vi "Configure ADCW.vi"(0 "VISA resource name":refnum<visa-resource-name>, 1 "Test Voltage (V)":string, 2 "Ramp Time (s)":string, 3 "Dwell Time (s)":string, 4 "Min Leakag (A)":string, 5 "Max Leakage (A)":string, 6 "DUT Type I":string(combo)="Isolated DUT", 7 "error in (no error)":errorcluster, 8 "Test Mode":string(combo)="ACW", 9 "DUT Type II (DCW Only)":string(combo)="Resistive DUT", 11 "Command Terminator":bool=TRUE) -> (20 "VISA resource name out":refnum<visa-resource-name>, 21 "Command Output":string, 25 "Error Message":string, 26 "Error Code":i32, 27 "error out":errorcluster)   [LabVIEW 2010, in "VITREK V7X.lvlib"]
doc: "Configures the <b>ACW</b> or <b>DCW</b> input.\n\n<b>Note:</b> please refer to the instrument manual for the <b>ACW/DCW</b> input specification."
uses:
  VITREK V7X.lvlib
panel:
  # "Yes\n\nNo"
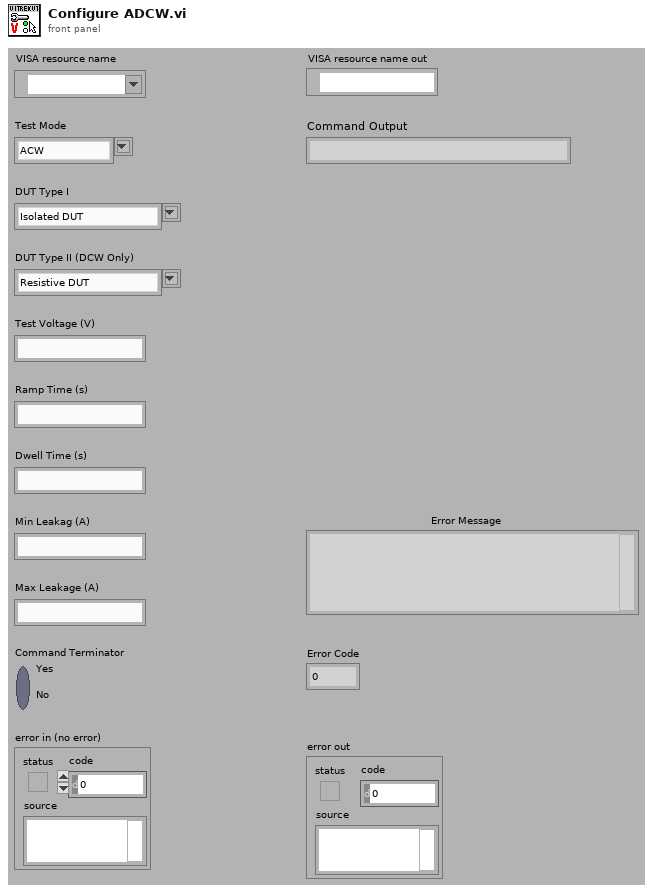
[diagram p1: front panel]
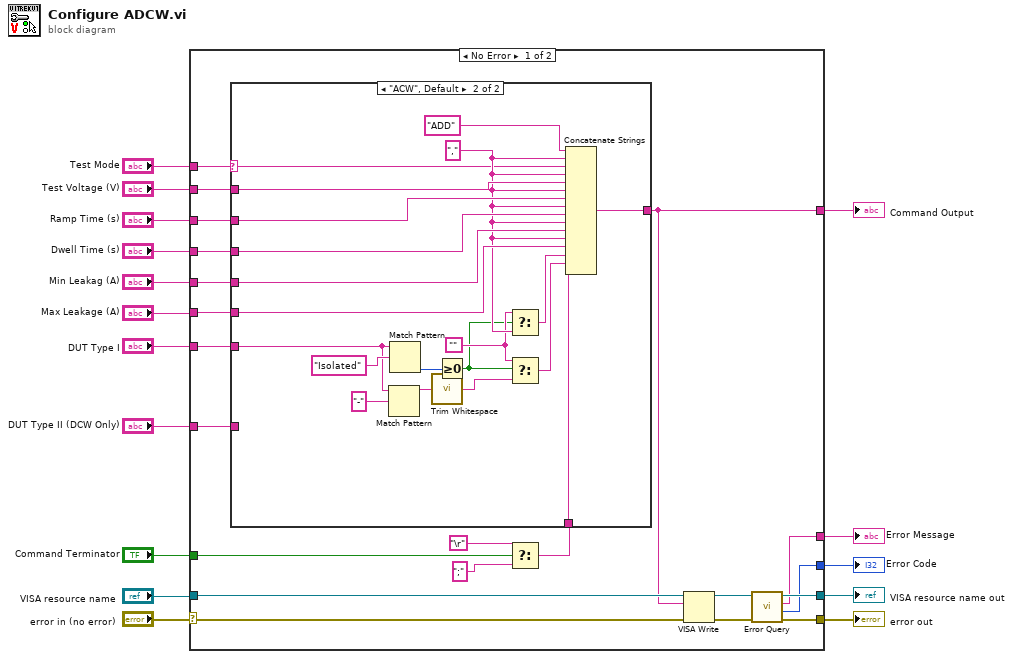
[diagram p0: block diagram]
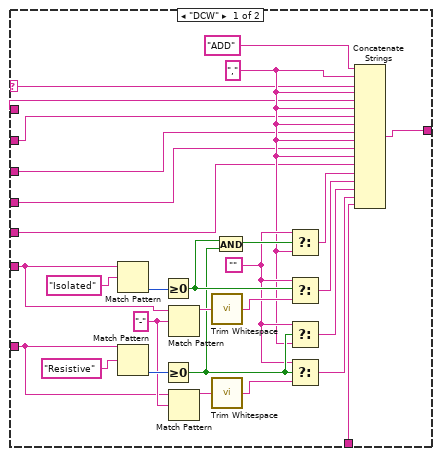
[diagram p2: hidden frame]
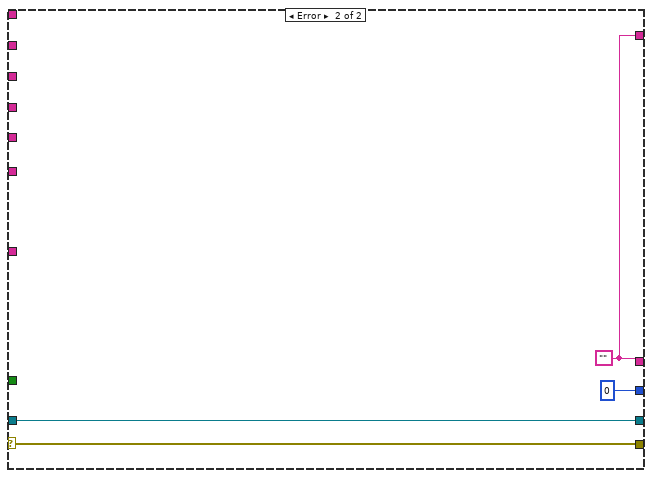
[diagram p3: hidden frame]
diagram:
  n1 = case shown="No Error" "error in (no error)" {
    selector: "error in (no error)" -> [w33 w89]
    tunnel: "VISA resource name" -> [w37 w90]
    tunnel: [w27 w87] -> w15
    tunnel: [w34 w90] -> w14
    tunnel: [w19 w89] -> w13
    tunnel: "Test Voltage (V)" -> [w32 _]
    tunnel: "Ramp Time (s)" -> [w31 _]
    tunnel: "Dwell Time (s)" -> [w30 _]
    tunnel: "Min Leakag (A)" -> [w29 _]
    tunnel: "Max Leakage (A)" -> [w28 _]
    tunnel: "Command Terminator" -> [w26 _]
    tunnel: "Test Mode" -> [w21 _]
    tunnel: "DUT Type I" -> [w22 _]
    tunnel: "DUT Type II (DCW Only)" -> [w20 _]
    tunnel: [w18 0 ("Error Code")] -> w2
    tunnel: [w17 w87] -> w1
    frame No Error {
      n2 = Select(t="\r", s=w26, f=";") -> (s? t:f=w23:string)
      n3 = case shown="\"ACW\", Default" w21 {
        selector: w21 -> [w47 w67]
        tunnel: w32 -> [w46 w86]
        tunnel: w31 -> [w45 w85]
        tunnel: w30 -> [w44 w84]
        tunnel: w29 -> [w43 w83]
        tunnel: w28 -> [w42 w82]
        tunnel: [w38 w80] -> w27
        tunnel: w23 -> [w39 w75]
        tunnel: w22 -> [w41 w70]
        tunnel: w20 -> [w40 _]
        frame "DCW" {
          w48 = "-"
          w51 = ""
          w50 = ","
          n4 = Match Pattern(string=w41, regular expression="Isolated") -> (offset past match=w62:i32)  [unwired: 1 in, 3 out]
          n5 = Match Pattern(string=w40, regular expression="Resistive") -> (offset past match=w58:i32)  [unwired: 1 in, 3 out]
          n6 = Greater Or Equal To 0?(x=w62) -> (x >= 0?=w55:bool)
          n7 = Greater Or Equal To 0?(x=w58) -> (x >= 0?=w52:bool)
          n8 = Match Pattern(string=w41, regular expression=w48) -> (before substring=w61:string)  [unwired: 1 in, 3 out]
          n9 = Match Pattern(string=w40, regular expression=w48) -> (before substring=w57:string)  [unwired: 1 in, 3 out]
          n10 = call <vilib>:"Trim Whitespace.vi"("string"=w61) -> ("trimmed string"=w60:string)  [unwired: 1 in]
          n11 = call <vilib>:"Trim Whitespace.vi"("string"=w57) -> ("trimmed string"=w56:string)  [unwired: 1 in]
          n12 = And(x=w55, y=w52) -> (x .and. y?=w54:bool)
          n13 = Select(t=w51, s=w54, f=w50) -> (s? t:f=w64:string)
          n14 = Select(t=w51, s=w55, f=w60) -> (s? t:f=w65:string)
          n15 = Select(t=w51, s=w52, f=w50) -> (s? t:f=w49:string)
          n16 = Select(t=w51, s=w52, f=w56) -> (s? t:f=w53:string)
          n17 = Concatenate Strings("ADD", w50, w47, w50, w46, w50, w45, w50, w44, w50, w43, w50, w42, w64, w65, w49, w53, w39) -> (w38:string)
        }
        frame "ACW", Default {
          w76 = ""
          w78 = ","
          n18 = Match Pattern(string=w70, regular expression="-") -> (before substring=w69:string)  [unwired: 1 in, 3 out]
          n19 = Match Pattern(string=w70, regular expression="Isolated") -> (offset past match=w73:i32)  [unwired: 1 in, 3 out]
          n20 = call <vilib>:"Trim Whitespace.vi"("string"=w69) -> ("trimmed string"=w68:string)  [unwired: 1 in]
          n21 = Greater Or Equal To 0?(x=w73) -> (x >= 0?=w72:bool)
          n22 = Select(t=w76, s=w72, f=w78) -> (s? t:f=w77:string)
          n23 = Select(t=w76, s=w72, f=w68) -> (s? t:f=w79:string)
          n24 = Concatenate Strings("ADD", w78, w67, w78, w86, w78, w85, w78, w84, w78, w83, w78, w82, w77, w79, w75) -> (w80:string)
        }
      }
      n25 = VISA Write(VISA resource name=w37, write buffer=w27, error in (no error)=w33) -> (VISA resource name out=w36:refnum<visa-resource-name>, error out=w35:errorcluster)  [unwired: 1 out]
      n26 = call "Error Query.vi"("error in (no error)"=w35, "VISA resource name"=w36) -> ("error out"=w19:errorcluster, "Error Code"=w18:i32, "Error Message"=w17:string, "VISA resource name out"=w34:refnum<visa-resource-name>)  [unwired: 6 in]
    }
    frame Error {
      w87 = ""
    }
  }
  "VISA resource name out" <- w14
  "error out" <- w13
  "Command Output" <- w15
  "Error Code" <- w2
  "Error Message" <- w1
